vi "set_Al_cond.vi"(0 "Aluminum Flow":dbl, 1 "Al Run":bool, 2 "Al Bubbler":bool, 3 "Al Active":bool) -> ()   [LabVIEW 2011]
uses:
  editor_lib/Flow_Globals.vi
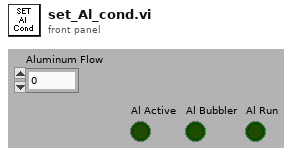
[diagram p1: front panel]
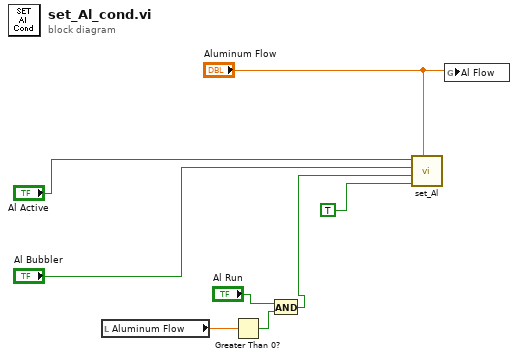
[diagram p0: block diagram]
diagram:
  n1 = local read "Aluminum Flow"() -> (w5:dbl)
  n2 = Greater Than 0?(x=w5) -> (x > 0?=w3:bool)
  n3 = And(x="Al Run", y=w3) -> (x .and. y?=w2:bool)
  n4 = call "set_Al.vi"("Aluminum Flow"="Aluminum Flow", "Al Remote"=TRUE, "Al Run"=w2, "Al Bubbler"="Al Bubbler", "Al Active"="Al Active") -> ()  [unwired: 5 in]
  n5 = global write "Flow_Globals.vi" "Al Flow"("Aluminum Flow") -> ()
